vi "Elapsed Timer (seconds).vi"(10 "time to Elapse (Minutes)":dbl=1.0 min=1.0 max=60.0 step=1.0, 11 "Reset":bool) -> (3 "Time has Elapsed":bool)   [LabVIEW 2011]
doc: "This VI uses the CPU clock to determine when a specified number of Minutes have gone by and trigger a true value. After a true value is output the clock resets to state when the next amount of specified time has elapsed. The count can be reset at any time by the user by specifying a true value in the reset input. Values can be 1 min to 60 min."
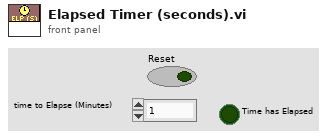
[diagram p1: front panel]
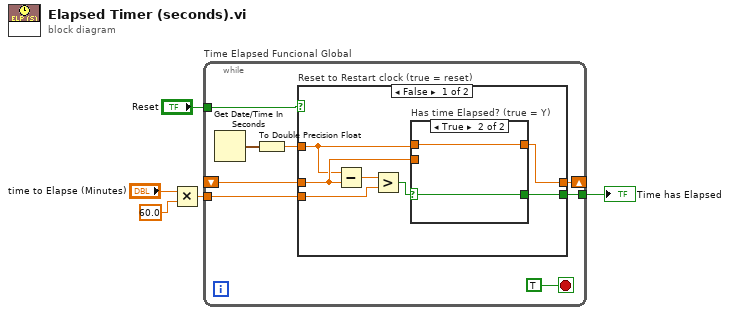
[diagram p0: block diagram]
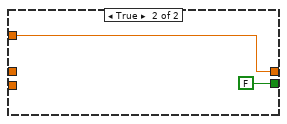
[diagram p3: hidden frame]
diagram:
  n1 = Multiply(x="time to Elapse (Minutes)", y=60.0) -> (x*y=w4:dbl)
  n2 = while "Time Elapsed Funcional Global" {
    tunnel: w4 -> [w13]
    shift-right: [w11] -> _
    shift-left: _ -> [w12]
    tunnel: [w7] -> w1
    tunnel: "Reset" -> [w6]
    stop <- TRUE stop-if-true
    n3 = Get Date/Time In Seconds() -> (seconds since 1Jan1904=w10:timestamp)
    n4 = To Double Precision Float(number=w10) -> (double precision float=w9:dbl)
    n5 = case "Reset to Restart clock (true = reset)" shown="False" w6 {
      tunnel: w13 -> [w20 _]
      tunnel: w12 -> [w18 _]
      tunnel: [w17 w26] -> w11
      tunnel: w9 -> [w16 w26]
      tunnel: [w14 FALSE] -> w7
      frame False {
        n6 = Subtract(x=w16, y=w18) -> (x-y=w19:dbl)
        n7 = Greater?(x=w19, y=w20) -> (0:w15:bool)
        n8 = case "Has time Elapsed? (true = Y)" shown="True" w15 {
          selector: w15 -> [w21 w23]
          tunnel: w16 -> [_ w24]
          tunnel: w18 -> [w22 _]
          tunnel: [w22 w24] -> w17
          tunnel: [w21 w23] -> w14
          frame False {
          }
          frame True {
          }
        }
      }
      frame True {
      }
    }
  }
  "Time has Elapsed" <- w1
